vi "array -- find monotonic segments -- testblock.vi"(9 "prev":dbl, 10 "next":dbl, 11 "up|dowm IN":enum16{"up", "down"}(ring)) -> (0 "dir change":bool, 3 "up|dowm OUT":enum16{"up", "down"}(ring))   [LabVIEW 2015]
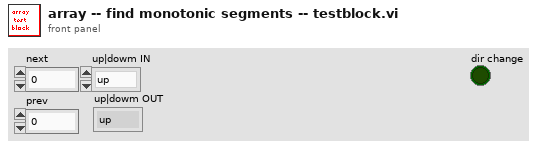
[diagram p1: front panel]
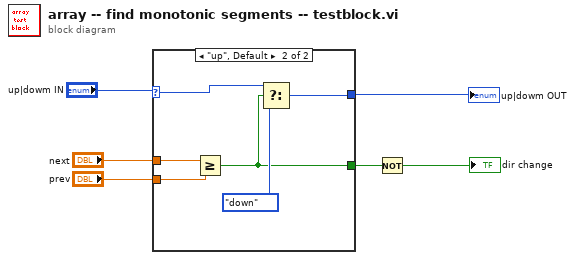
[diagram p0: block diagram]
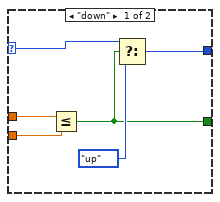
[diagram p2: hidden frame]
diagram:
  n1 = case shown="\"up\", Default" "up|dowm IN" {
    selector: "up|dowm IN" -> [w10 w16]
    tunnel: "next" -> [w12 w18]
    tunnel: "prev" -> [w11 w17]
    tunnel: [w8 w14] -> w3
    tunnel: [w7 w13] -> w2
    frame "down" {
      n2 = Less Or Equal?(x=w12, y=w11) -> (x <= y?=w7:bool)
      n3 = Select(t=w10, s=w7, f=enum16{"up", "down"}."up") -> (s? t:f=w8:enum16{"up", "down"})
    }
    frame "up", Default {
      n4 = Greater Or Equal?(x=w18, y=w17) -> (x >= y?=w13:bool)
      n5 = Select(t=w16, s=w13, f=enum16{"up", "down"}."down") -> (s? t:f=w14:enum16{"up", "down"})
    }
  }
  "up|dowm OUT" <- w3
  n6 = Not(x=w2) -> (.not. x?=→"dir change":bool)
